vi "CC Script Generate Channels.vi"(8 "error in (no error)":errorcluster) -> (0 "error out":errorcluster, 2 "Channel Names":string[](array[string])=["Telescope RA", "Telescope DEC", "Telescope Moving?", "Telescope Status"], 3 "Channel List":refnum<class "HK Item.lvclass">[](array[class]))   [LabVIEW 2021]
uses:
  hk-channel-class/HK Item/HK Item.lvclass
  hk-channel-class/HK Item/HK Channel Units and Setup.ctl
  hk-channel-class/HK Item/HK Channel enum Data Type.ctl
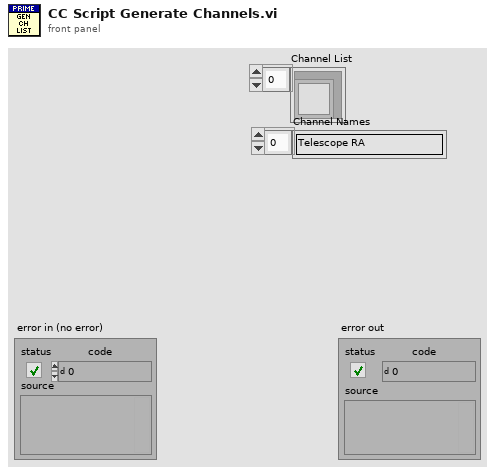
[diagram p1: front panel]
types:
  T1 = typedef "HK Item.lvclass/HK Channel Units and Setup.ctl" = cluster{"Unit Type":string, "Units":string, "Configuration":string, "Digits":i32, "Data Type":T2, "Exponential?":bool, "Source":string}
  T2 = typedef "HK Item.lvclass/HK Channel enum Data Type.ctl" = enum16{"Floating Point", "Integer", "Enum", "String", "Waveform", "File"}
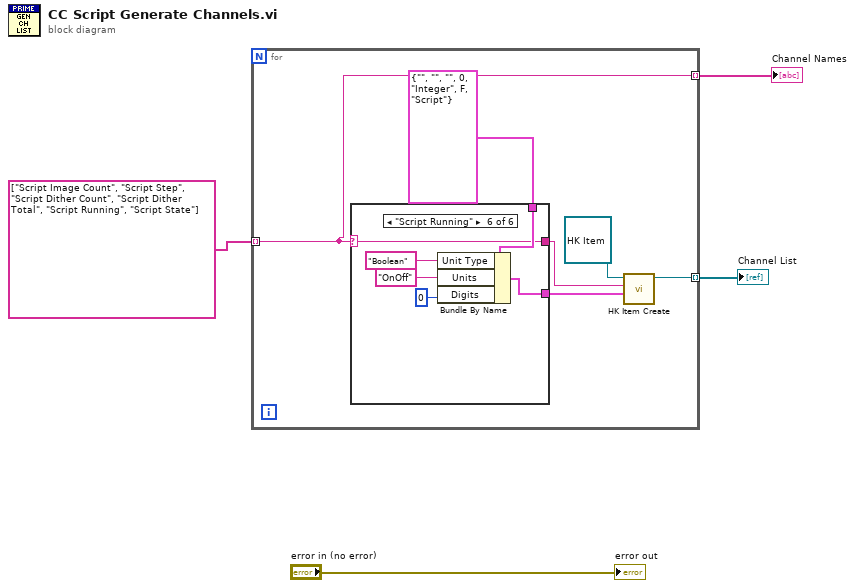
[diagram p0: block diagram]
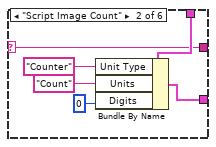
[diagram p3: hidden frame]
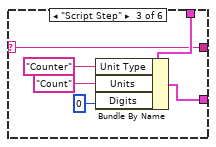
[diagram p4: hidden frame]
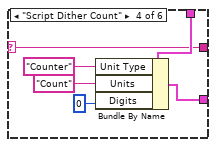
[diagram p5: hidden frame]
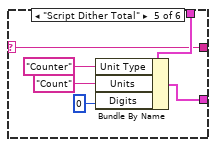
[diagram p6: hidden frame]
diagram:
  n1 = for {
    tunnel: string[] ["Script Image Count", "Script Step", "Script Dither Count", "Script Dither Total", "Script Running", "Script State"] -> [w5] mode=indexing
    tunnel: [w7] -> w3 mode=indexing
    tunnel: [w5] -> w2 mode=indexing
    n2 = case shown="\"Script Running\"" w5 {
      selector: w5 -> [w12 w13 w19 w25 w31 w37]
      tunnel: T1 {"Unit Type"="", "Units"="", "Configuration"="", "Digits"=0, "Data Type"=enum."Integer", "Exponential?"=FALSE, "Source"="Script"} ("Channel Setup") -> [w11 w18 w24 w30 w36 w42]
      tunnel: [w11 w14 w20 w26 w32 w38] -> w10
      tunnel: [w12 w13 w19 w25 w31 w37] -> w9
      frame "False", Default {
      }
      frame "Script Image Count" {
        n3 = Bundle By Name(cluster=w18, "Unit Type"="Counter", "Units"="Count", "Digits"=0) -> (w14:T1)
      }
      frame "Script Step" {
        n4 = Bundle By Name(cluster=w24, "Unit Type"="Counter", "Units"="Count", "Digits"=0) -> (w20:T1)
      }
      frame "Script Dither Count" {
        n5 = Bundle By Name(cluster=w30, "Unit Type"="Counter", "Units"="Count", "Digits"=0) -> (w26:T1)
      }
      frame "Script Dither Total" {
        n6 = Bundle By Name(cluster=w36, "Unit Type"="Counter", "Units"="Count", "Digits"=0) -> (w32:T1)
      }
      frame "Script Running" {
        n7 = Bundle By Name(cluster=w42, "Unit Type"="Boolean", "Units"="OnOff", "Digits"=0) -> (w38:T1)
      }
    }
    n8 = call-dynamic "HK Item Create.vi"("Channel Setup"=w10, "Name"=w9, "HK Item in"=refnum<class "HK Item.lvclass"> refnum) -> ("HK Item out"=w7:refnum<class "HK Item.lvclass">)  [unwired: 7 in, 1 out]
  }
  "Channel List" <- w3
  "Channel Names" <- w2
  "error out" <- "error in (no error)"
